vi "Prepare Bus Monitor Interface.vi"(9 "Datum Name":string, 11 "IBusMonitor":refnum<class "IBusMonitor.lvclass">) -> (2 "Valid Transport":refnum<class "ITransport.lvclass">, 3 "SubscriptionPolicy":refnum<class "ISubscriptionPolicy.lvclass">)   [LabVIEW 2018, in "MVA Framework.lvlib" / "MonitoredMediator.lvlib" / "IBusMonitor.lvclass"]
doc: "抽象方法\n准备总线监视器接口"
uses:
  IBusMonitor.lvclass
  IMediator/ISubscriptionPolicy/ISubscriptionPolicy.lvclass
  composed-transport/Source/ITransport/ITransport.lvclass
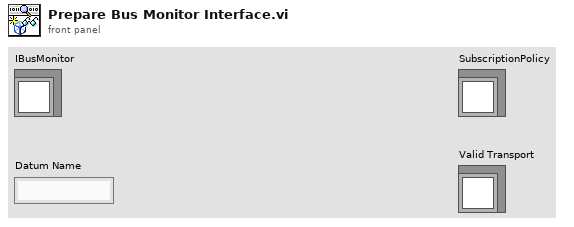
[diagram p1: front panel]
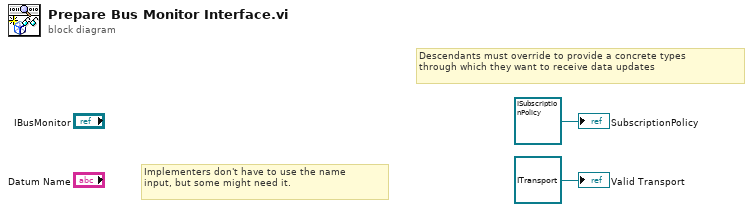
[diagram p0: block diagram]
diagram:
  # "Implementers don't have to use the name\ninput, but some might need it."
  # "Descendants must override to provide a concrete types\nthrough which they want to receive data updates"
  "Valid Transport" <- refnum<class "ITransport.lvclass"> refnum ("Notification Msg Type")
  "SubscriptionPolicy" <- refnum<class "ISubscriptionPolicy.lvclass"> refnum ("Bus Monitor SubscriptionPolicy")
